vi "FP_Get Pane.vi"(8 "Error":errorcluster, 9 "Pane Index":i32, 11 "VI":refnum<vi>) -> (0 "Error Out":errorcluster, 2 "Pane Refnum Out":refnum<vi>, 3 "VI Out":refnum<vi>)   [LabVIEW 2020]
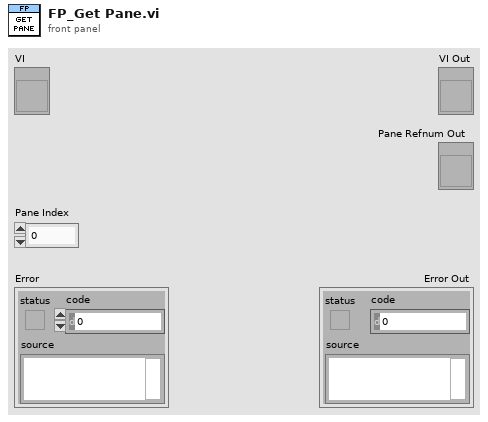
[diagram p1: front panel]
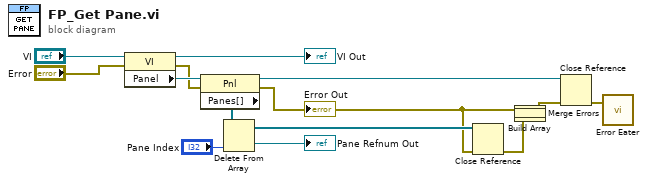
[diagram p0: block diagram]
diagram:
  n1 = property class="VI"(reference="VI", error in="Error") -> (reference out=→"VI Out":refnum<vi>, error out=w7:errorcluster, "Panel"=w9:refnum<vi>)
  n2 = property class="Pnl"(reference=w9, error in=w7) -> (reference out=w10:refnum<vi>, error out=w2:errorcluster, "Panes[]"=w8:refnum<vi>[])
  "Error Out" <- w2
  n3 = Delete From Array(array=w8, index="Pane Index") -> (deleted portion=→"Pane Refnum Out":refnum<vi>, array with subset deleted=w6:refnum<vi>[])  [unwired: 1 in]
  n4 = Close Reference(reference=w6, error in (no error)=w2) -> (error out=w4:errorcluster)
  n5 = Build Array(w2, w4) -> (w1:errorcluster[])
  n6 = Merge Errors(w1) -> (w3:errorcluster)
  n7 = Close Reference(reference=w10, error in (no error)=w3) -> (error out=w5:errorcluster)
  n8 = call "Error Eater.vi"("error in (no error)"=w5) -> ()  [unwired: 2 in]
